vi "Subvi wait and shoot.vi"(8 "Stop":bool, 9 "Start":bool) -> (1 "Output":bool)   [LabVIEW 2017]
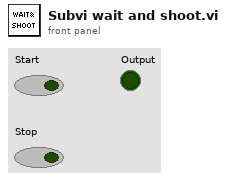
[diagram p1: front panel]
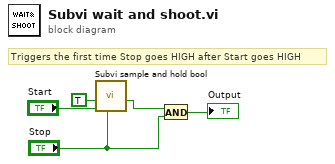
[diagram p0: block diagram]
diagram:
  # "Triggers the first time Stop goes HIGH after Start goes HIGH"
  n1 = call "Subvi sample and hold bool.vi"("Reset"="Stop", "Refresh"="Start", "Input"=TRUE) -> ("Output"=w5:bool)  [unwired: 8 in]
  n2 = And(x=w5, y="Stop") -> (x .and. y?=→"Output":bool)
